vi "ExamenD_ProblemaUltimo.vi"() -> ()   [LabVIEW 2024]
panel:
  out "Mensaje de temperatura":string
  out "Indicador Rango":bool
  out "Numeric":i32
  in  "stop":bool
  out "Grafica de temperaturas":dynamicdata(graph)
  # "Valor de temperatura"
  # "grados,           de rango"
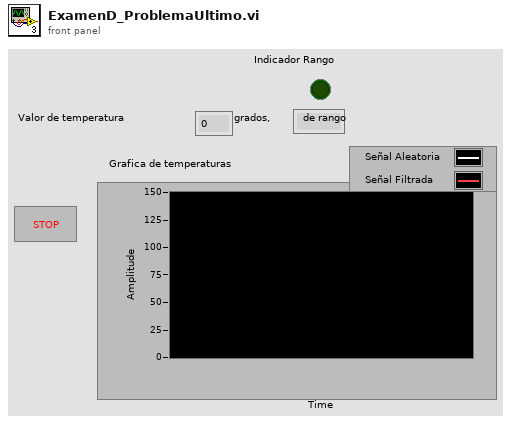
[diagram p1: front panel]
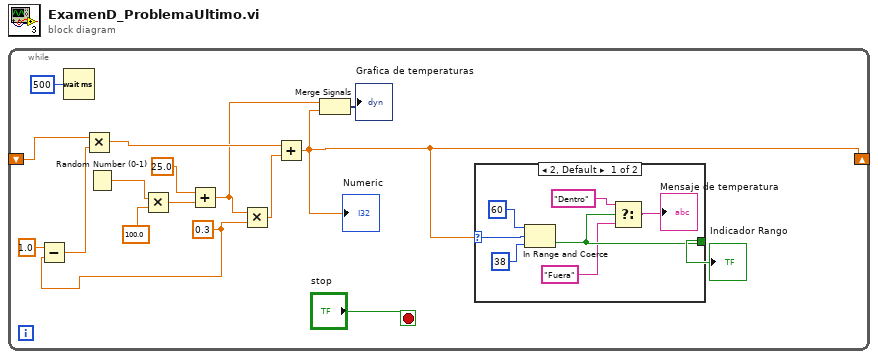
[diagram p0: block diagram]
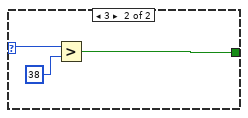
[diagram p2: hidden frame]
diagram:
  n1 = while {
    shift-right: [w2] -> _
    shift-left: _ -> [w13]
    stop <- "stop" stop-if-true
    w14 = 0.3 ("y")
    n2 = Subtract(x=1.0, y=w14) -> (x-y=w12:dbl)
    n3 = Wait (ms)(milliseconds to wait=u32 500) -> ()  [unwired: 1 out]
    n4 = Multiply(x=w13, y=w12) -> (x*y=w11:dbl)
    n5 = Random Number (0-1)() -> (number: 0 to 1=w7:dbl)
    n6 = Multiply(x=w7, y=100.0) -> (x*y=w8:dbl)
    n7 = Add(x=25.0, y=w8) -> (x+y=w3:dbl)
    n8 = Multiply(x=w3, y=w14) -> (x*y=w5:dbl)
    n9 = Add(x=w11, y=w5) -> (x+y=w2:dbl)
    "Numeric" <- w2
    n10 = Merge Signals(w3, w2) -> (→"Grafica de temperaturas":dynamicdata)
    n11 = case shown="2, Default" w2 {
      selector: w2 -> [w23 w26]
      tunnel: [w20 w24] -> w1
      frame 2, Default {
        n12 = In Range and Coerce(upper limit=60, x=w23, lower limit=38) -> (In Range?=w20:bool)  [unwired: 1 out]
        n13 = Select(t="Dentro", s=w20, f="Fuera") -> (s? t:f=→"Mensaje de temperatura":string)
      }
      frame 3 {
        n14 = Greater?(x=w26, y=38) -> (0:w24:bool)
      }
    }
    "Indicador Rango" <- w1
  }
